vi "ATSh_GetCPLDVersion.vi"(11 "HandleIn":u32) -> (0 "Return Code":u32, 1 "Board":string, 2 "Version":string, 3 "HandleOut":u32, 4 "ID":i32)   [LabVIEW 2010]
doc: "_____AlazarTech, Scope_____\n\nRetrieve the CPLG version number.\n\nInput:\n\"HandleIn\" = device to retrieve information\n\nOutput:\n\"HandleOut\" = device information\n\"Version\" = version\n\"Board\" = board name\n\"ID\" = board identification"
uses:
  ATS_ctl/ATS_Cards_GBL.vi
  ATSApi.dll
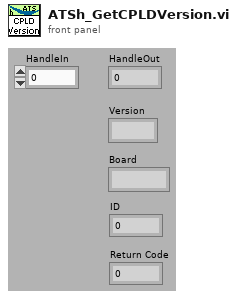
[diagram p1: front panel]
types:
  T1 = typedef "ATS_Global_Specs_Ctrl.ctl" = cluster{"ClckSource":cluster{"Internal":bool, "External":bool, "Medium Ext.":bool, "Slow Ext.":bool, "Ext. AC":bool, "Ext. DC":bool, "Ext. (PLL)":bool}, "ClckRate":cluster{"1 kS/s":bool, "2 kS/s":bool, "5 kS/s":bool, "10 kS/s":bool, "20 kS/s":bool, "50 kS/s":bool, "100 kS/s":bool, "200 kS/s":bool, "500 kS/s":bool, "1 MS/s":bool, "2 MS/s":bool, "5 MS/s":bool, "10 MS/s":bool, "20 MS/s":bool, "25 MS/s":bool, "50 MS/s":bool, "100 MS/s":bool, "125 MS/s":bool, "160 MS/s":bool, "180 MS/s":bool, "200 MS/s":bool, "250 MS/s":bool, "500 MS/s":bool, "1 GS/s":bool}, "ClckEdge":cluster{"Rising":bool, "Falling":bool}, "InputCoupling":cluster{"AC":bool, "DC":bool}, "InputRange":cluster{"20mV":bool, "40mV":bool, "50mV":bool, "80mV":bool, "100mV":bool, "200mV":bool, "400mV":bool, "500mV":bool, "800mV":bool, "1 V":bool, "2 V":bool, "4 V":bool, "5 V":bool, "8 V":bool, "10 V":bool, "16 V":bool, "20 V":bool, "40 V":bool, "HiFi":bool, "1.25 V":bool}, "Impedance":cluster{"1M ohms":bool, "50 ohms":bool, "300 ohms":bool}, "Bandwidth":cluster{"Full":bool, "Reduce":bool}, "RangeLim(50)":string, "AsyncDMA":cluster{"OnBoard":bool, "FPGA":bool}, "Memory":cluster{"VerifMem":bool, "HighMem":bool, "Combine":bool, "HighRecord":bool}, "ExtTrigCoupling":cluster{"AC":bool, "DC":bool}, "ExtTrigRange":cluster{"1 V":bool, "5 V":bool, "\nTTL":bool}, "AUX_IO_Trig":cluster{"Trig_Out":bool, "Trig_In":bool}, "AUX_IO_Slope":cluster{"Rising":bool, "Falling":bool}, "MaxPretrig":cluster{"MEM":u32, "FIFO":u32}, "AUX_I/O_Trig":cluster{"OUT_Trigger":bool, "OUT_PACER":bool, "OUT_BUSY":bool, "OUT_CLOCK":bool, "OUT_RESERVED":bool, "OUT_CAPTURE_ALMOST_DONE":bool, "OUT_AUXILIARY":bool, "OUT_SERIAL_DATA":bool, "IN_TRIGGER_ENABLE":bool, "IN_DIGITAL_TRIGGER":bool, "IN_GATE":bool, "IN_CAPTURE_ON_DEMAND":bool, "IN_RESET_TIMESTAMP":bool, "IN_SLOW_EXTERNAL_CLOCK":bool, "INPUT_AUXILIARY":bool, "INPUT_SERIAL_DATA":bool}, "ChannelsPerBoard":u8}
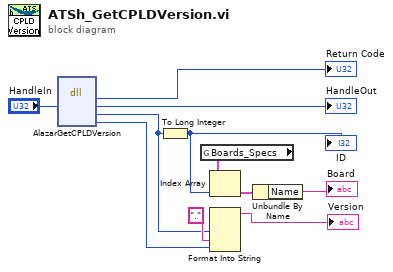
[diagram p0: block diagram]
diagram:
  n1 = dll-call lib="ATSApi.dll" fn="AlazarGetCPLDVersion"("h"="HandleIn") -> (→"Return Code":u32, "h"=→"HandleOut":u32, "Major"=w4:u8, "Minor"=w8:u8)  [unwired: 5 in, 2 out]
  n2 = To Long Integer(number=w4) -> (32bit integer=w5:i32)
  "ID" <- w5
  n3 = global read "ATS_Cards_GBL.vi" "Boards_Specs"() -> (w1:cluster{"Name":string, "Specifications":T1}[])
  n4 = Index Array(array=w1, index=w5) -> (element=w3:cluster{"Name":string, "Specifications":T1})
  n5 = Format Into String(w4, ".", w8) -> (resulting string=→"Version":string)  [unwired: 3 in, 1 out]
  n6 = Unbundle By Name(w3) -> ("Name"=→"Board":string)
